vi "Obtain Session.vi"   [LabVIEW 2012, in "REx.lvlib" / "Remote Connection Session.lvclass"]
uses:
  Remote Connection Session.lvclass
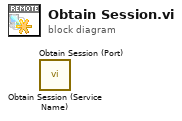
[diagram p0: block diagram]
diagram:
  n1 = call "Obtain Session (Service Name).vi"() -> ()  [unwired: 13 in, 3 out]
  n2 = call "Obtain Session (Port).vi"() -> ()  [unwired: 13 in, 3 out]
